vi "Read Azimuth Settings.vi"(8 "error in (no error)":errorcluster, 11 "LiDAR in":refnum<class "LiDAR.lvclass">) -> (0 "error out":errorcluster, 2 "Azimuth":cluster{"Min >=-60":dbl, "Max <=+60 ":dbl}, 3 "LiDAR out":refnum<class "LiDAR.lvclass">)   [LabVIEW 2018]
uses:
  LiDAR.lvclass
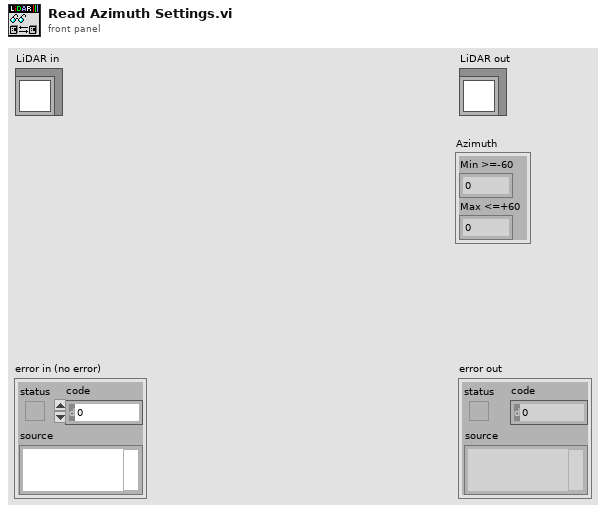
[diagram p1: front panel]
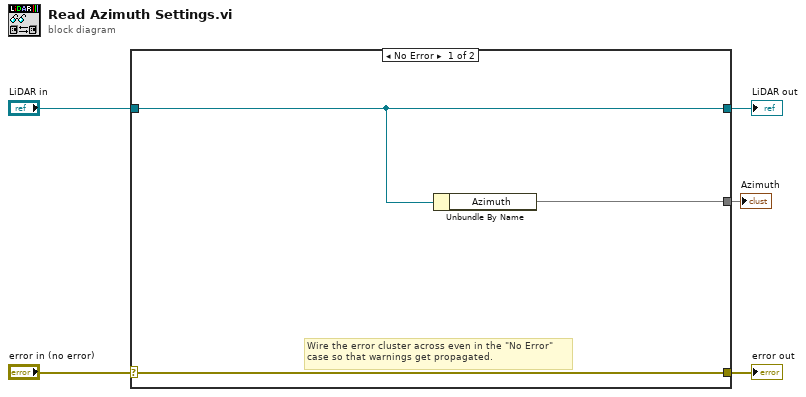
[diagram p0: block diagram]
diagram:
  n1 = case shown="No Error" "error in (no error)" {
    selector: "error in (no error)" -> [w8 w10]
    tunnel: [w8 w10] -> w4
    tunnel: [w7 w9] -> w2
    tunnel: "LiDAR in" -> [w7 w9]
    tunnel: [w6 _] -> w1
    frame No Error {
      # "Wire the error cluster across even in the \"No Error\"\ncase so that warnings get propagated."
      n2 = Unbundle By Name(w7) -> ("Azimuth"=w6)
    }
    frame Error {
    }
  }
  "error out" <- w4
  "LiDAR out" <- w2
  "Azimuth" <- w1
